vi "Get_process_notifications.vi"(11 "Notifier Refnums":refnum<notifier>[](array[refnum])) -> (3 "Notifications out":string[](array[string]))   [LabVIEW 2017, in "labview-standard-library.lvlib"]
uses:
  labview-standard-library.lvlib
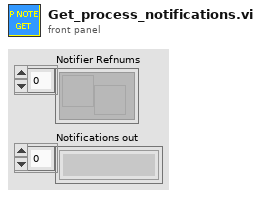
[diagram p1: front panel]
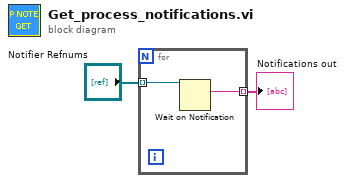
[diagram p0: block diagram]
diagram:
  n1 = for {
    tunnel: "Notifier Refnums" -> [w4] mode=indexing
    tunnel: [w3] -> w1 mode=indexing
    n2 = Wait on Notification(notifier=w4) -> (notification=w3:string)  [unwired: 3 in, 3 out]
  }
  "Notifications out" <- w1
